vi "Microgear_onAbsent.vi"(9 "lenght":u8, 10 "msg":string, 11 "topic":string) -> ()   [LabVIEW 2014]
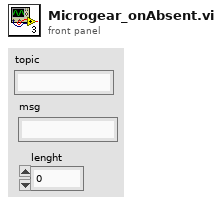
[diagram p1: front panel]
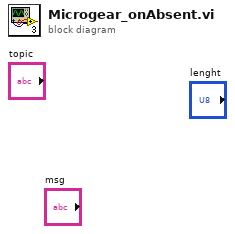
[diagram p0: block diagram]
diagram:
